vi "PercentCO2.vi"(2 "log fO2 rel. IW/IM":dbl, 3 "Temperature":dbl) -> (0 "Fugacity":dbl, 1 "%CO2":dbl)   [LabVIEW 2009]
uses:
  <vilib>/gmath/interp.llb/Interpolate 2D (1d xi,yi).vi
  <vilib>/Utility/file.llb/Read From Spreadsheet File (DBL).vi
  <vilib>/gmath/NI_Gmath.lvlib
panel:
  out "Array":dbl[][](array[numeric])
  out "CO2":dbl[][](array[numeric])
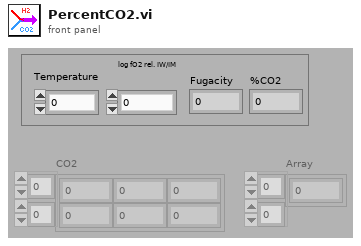
[diagram p1: front panel]
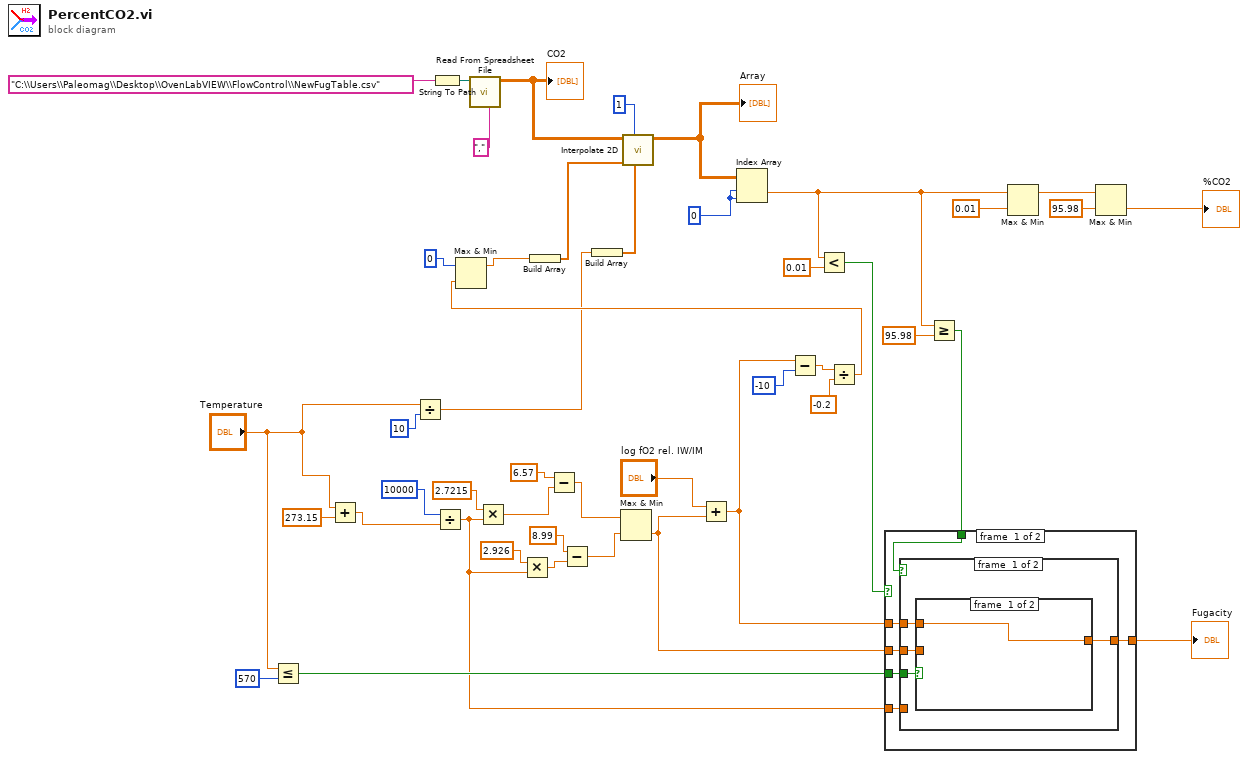
[diagram p0: block diagram]
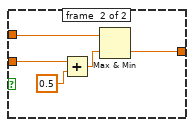
[diagram p2: hidden frame]
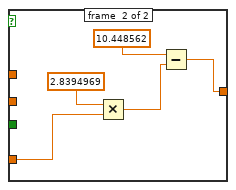
[diagram p3: hidden frame]
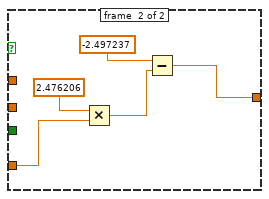
[diagram p4: hidden frame]
diagram:
  w30 = 0
  n1 = Less Or Equal?(x="Temperature", y=570) -> (x <= y?=w14:bool)
  n2 = Add(x="Temperature", y=273.15) -> (x+y=w40:dbl)
  n3 = Divide(x="Temperature", y=10) -> (x/y=w18:dbl)
  n4 = String To Path(string="C:\\Users\\Paleomag\\Desktop\\OvenLabVIEW\\FlowControl\\NewFugTable.csv" ("prompt (Open existing file)")) -> (path=w44:path)
  n5 = Divide(x=10000, y=w40) -> (x/y=w9:dbl)
  n6 = call-poly <vilib>:"Read From Spreadsheet File.vi"("delimiter (\\t)"=",", "file path (dialog if empty)"=w44) -> ("all rows"=w20:dbl[][])  [unwired: 5 in, 4 out]
  "CO2" <- w20
  n7 = Multiply(x=2.7215, y=w9) -> (x*y=w37:dbl)
  n8 = Multiply(x=2.926, y=w9) -> (x*y=w34:dbl)
  n9 = Subtract(x=6.57, y=w37) -> (x-y=w33:dbl)
  n10 = Subtract(x=8.99, y=w34) -> (x-y=w32:dbl)
  n11 = Build Array(w18) -> (w27:dbl[])
  n12 = Max & Min(x=w33, y=w32) -> (min(x,y)=w12:dbl)  [unwired: 1 out]
  n13 = Add(x="log fO2 rel. IW/IM", y=w12) -> (x+y=w13:dbl)
  n14 = Subtract(x=w13, y=-10) -> (x-y=w23:dbl)
  n15 = Divide(x=w23, y=-0.2) -> (x/y=w19:dbl)
  n16 = Max & Min(x=0, y=w19) -> (max(x,y)=w22:dbl)  [unwired: 1 out]
  n17 = Build Array(w22) -> (w28:dbl[])
  n18 = call-poly <vilib>:"Interpolate 2D.vi"("yi"=w27, "method"=1, "xi"=w28, "Z"=w20) -> ("zi"=w29:dbl[][])  [unwired: 4 in, 3 out]
  "Array" <- w29
  n19 = Index Array(array=w29, index (row)=w30, index (col)=w30) -> (element=w5:dbl)
  n20 = Less?(x=w5, y=0.01) -> (x < y?=w10:bool)
  n21 = Greater Or Equal?(x=w5, y=95.98) -> (x >= y?=w7:bool)
  n22 = case shown="True" w10 {
    tunnel: w14 -> [w51 _]
    tunnel: [w50 w69] -> w1
    tunnel: w13 -> [w49 _]
    tunnel: w12 -> [w48 _]
    tunnel: w9 -> [w46 w68]
    tunnel: w7 -> [w47 _]
    frame #0 {
      n23 = case shown="True" w47 {
        tunnel: w51 -> [w55 _]
        tunnel: [w54 w62] -> w50
        tunnel: w49 -> [w53 _]
        tunnel: w48 -> [w52 _]
        tunnel: w46 -> [_ w63]
        frame #0 {
          n24 = case shown="True" w55 {
            tunnel: [w56 w61] -> w54
            tunnel: w53 -> [w56 w60]
            tunnel: w52 -> [_ w58]
            frame #0 {
            }
            frame #1 {
              n25 = Add(x=w58, y=0.5) -> (x+y=w57:dbl)
              n26 = Max & Min(x=w60, y=w57) -> (min(x,y)=w61:dbl)  [unwired: 1 out]
            }
          }
        }
        frame #1 {
          n27 = Multiply(x=2.8394969, y=w63) -> (x*y=w65:dbl)
          n28 = Subtract(x=10.448562, y=w65) -> (x-y=w62:dbl)
        }
      }
    }
    frame #1 {
      n29 = Multiply(x=2.476206, y=w68) -> (x*y=w70:dbl)
      n30 = Subtract(x=-2.497237, y=w70) -> (x-y=w69:dbl)
    }
  }
  "Fugacity" <- w1
  n31 = Max & Min(x=w5, y=0.01) -> (max(x,y)=w6:dbl)  [unwired: 1 out]
  n32 = Max & Min(x=w6, y=95.98) -> (min(x,y)=→"%CO2":dbl)  [unwired: 1 out]
